vi "Coord window-Handle mouse click on map.vi"(9 "Button":u16, 11 "Coordinates of pixel clicked on":T1) -> ()   [LabVIEW 2020]
uses:
  <vilib>/Utility/miscctls.llb/LVPoint32TypeDef.ctl
  Globals/Coord window-Globals.vi
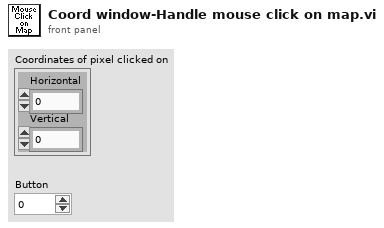
[diagram p1: front panel]
types:
  T1 = typedef "LVPoint32TypeDef.ctl" = cluster{"Horizontal":i32, "Vertical":i32}
  T2 = typedef "Coordinate list window refs.ctl" = cluster{"Window Name (i.e. Key)":string, "menu reference":refnum<k9>, "VI's reference":refnum<vi>, "Pane 1":refnum<vi>, "Pane 2":refnum<vi>, "Coord Listbox":refnum<vi>, "File name":refnum<vi>, "Picture Map":refnum<vi>, "Stage XYZ Position ind.":refnum<vi>}
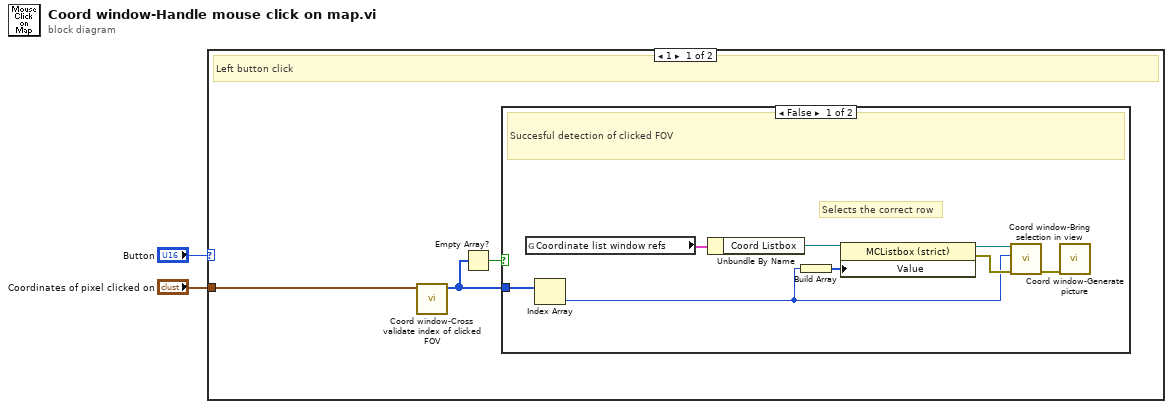
[diagram p0: block diagram]
diagram:
  n1 = case shown="1" "Button" {
    tunnel: "Coordinates of pixel clicked on" -> [w3 _]
    frame 1 {
      # "Left button click"
      n2 = call "Coord window-Cross validate index of clicked FOV.vi"("Coordinates of pixel clicked on"=w3) -> ("Output Array"=w4:i32[])  [unwired: 10 in]
      n3 = Empty Array?(array=w4) -> (empty?=w5:bool)
      n4 = case shown="False" w5 {
        tunnel: w4 -> [w13 _]
        frame False {
          # "Selects the correct row"
          # "Succesful detection of clicked FOV"
          n5 = global read "Coord window-Globals.vi" "Coordinate list window refs"() -> (w11:T2)
          n6 = Index Array(array=w13) -> (element=w7:i32)  [unwired: 1 in]
          n7 = Unbundle By Name(w11) -> ("Coord Listbox"=w10:refnum<vi>)
          n8 = Build Array(w7) -> (w12:i32[])
          n9 = property class="MCListbox (strict)"(reference=w10, "Value"=w12) -> (reference out=w9:refnum<vi>, error out=w8:errorcluster)  [unwired: 1 in]
          n10 = call "Coord window-Bring selection in view.vi"("error in (no error)"=w8, "Index of selected row"=w7, "MulticolumnListbox in"=w9) -> ("error out"=w6:errorcluster)  [unwired: 7 in, 1 out]
          n11 = call "Coord window-Generate picture.vi"("error in (no error)"=w6) -> ()  [unwired: 10 in, 1 out]
        }
        frame True {
          # "Could not detect which FOV the user clicked on"
        }
      }
    }
    frame Default {
      # "Not a left button click"
    }
  }
